vi "Do Turn.vi"(9 "Teams In":refnum<class "Team.lvclass">[](array[class]), 10 "Round":u32, 11 "Map in":refnum<class "Map.lvclass">) -> (1 "Teams":refnum<class "Team.lvclass">[](array[class]), 3 "Map out":refnum<class "Map.lvclass">, 4 "Turn Results":T1)   [LabVIEW 2020, in "SquareBattle.lvlib" / "Map.lvclass"]
uses:
  Map.lvclass
  Team/Team.lvclass
  Turn Results.ctl
  SquareBattle.lvlib
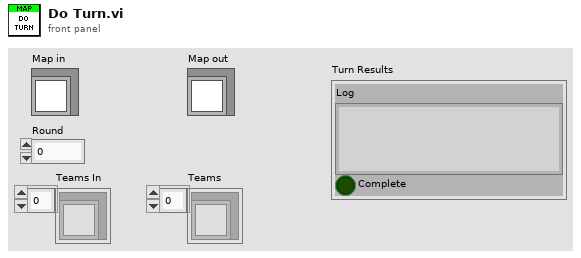
[diagram p1: front panel]
types:
  T1 = typedef "SquareBattle.lvlib/Turn Results.ctl" = cluster{"Log":string, "Complete":bool}
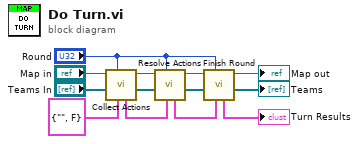
[diagram p0: block diagram]
diagram:
  n1 = call "Collect Actions.vi"("Turn Results In"=T1 {"Log"="", "Complete"=FALSE}, "Round"="Round", "Teams In"="Teams In", "Map in"="Map in") -> ("Teams"=w9:refnum<class "Team.lvclass">[], "Map out"=w10:refnum<class "Map.lvclass">, "Turn Results"=w8:T1)  [unwired: 5 in]
  n2 = call "Resolve Actions.vi"("Turn Results In"=w8, "Round"="Round", "Teams In"=w9, "Map in"=w10) -> ("Teams"=w5:refnum<class "Team.lvclass">[], "Map out"=w7:refnum<class "Map.lvclass">, "Turn Results"=w4:T1)  [unwired: 5 in]
  n3 = call "Finish Round.vi"("Turn Results In"=w4, "Round"="Round", "Teams In"=w5, "Map in"=w7) -> ("Teams"=→"Teams":refnum<class "Team.lvclass">[], "Map out"=→"Map out":refnum<class "Map.lvclass">, "Turn Results"=→"Turn Results":T1)  [unwired: 5 in]
